vi "Create.vi"(8 "error in":errorcluster, 11 "LUT":variant) -> (0 "error out":errorcluster, 3 "ORM_lib.lvlib:ObjectLUT.lvclass":refnum<class "ObjectLUT.lvclass">)   [LabVIEW 2020, in "ORM_lib.lvlib" / "ObjectLUT.lvclass"]
uses:
  ObjectLUT.lvclass
  ObjectLUT.lvclass/ObjectLUT.ctl
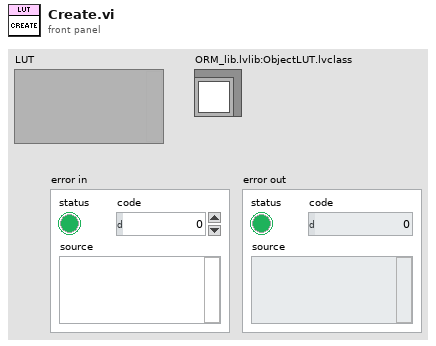
[diagram p1: front panel]
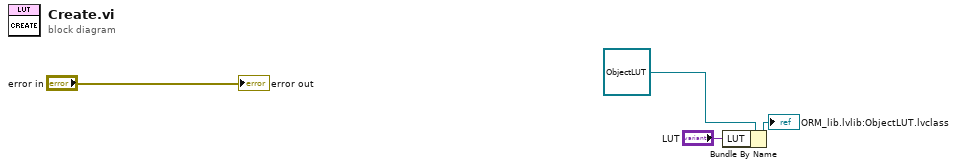
[diagram p0: block diagram]
diagram:
  n1 = Bundle By Name(cluster=refnum<class "ObjectLUT.lvclass"> refnum ("ORM_lib.lvlib:ObjectLUT.lvclass"), "LUT"="LUT") -> (→"ORM_lib.lvlib:ObjectLUT.lvclass":refnum<class "ObjectLUT.lvclass">)
  "error out" <- "error in"
